vi "NATS SUB.vi"(6 "timeout ms (conn default)":i32=-2, 7 "queue group":string, 8 "error in":errorcluster caption="error in (no error)", 9 "subject":string, 10 "sub id":string, 11 "nats connection in":T1={"connection ID"=refnum, "server INFO"="", "timeout ms"=5000, "verbose?"=FALSE, "server headers?"=FALSE, "client headers?"=FALSE}) -> (0 "error out":errorcluster, 2 "dup sub id":string, 3 "dup nats connection":T1={"connection ID"=refnum, "server INFO"="", "timeout ms"=5000, "verbose?"=FALSE, "server headers?"=FALSE, "client headers?"=FALSE})   [LabVIEW 2013, in "NATS Core.lvlib"]
doc: "Subscribes to a NATS subject with the specified subscription ID."
uses:
  NATS Core.lvlib
  Controls/nats connection.ctl
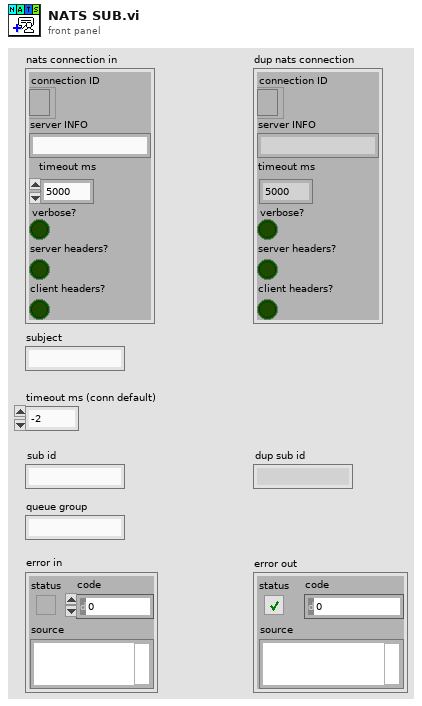
[diagram p1: front panel]
types:
  T1 = typedef "NATS Core.lvlib/nats connection.ctl" = cluster{"connection ID":refnum<k5>, "server INFO":string, "timeout ms":i32, "verbose?":bool, "server headers?":bool, "client headers?":bool}
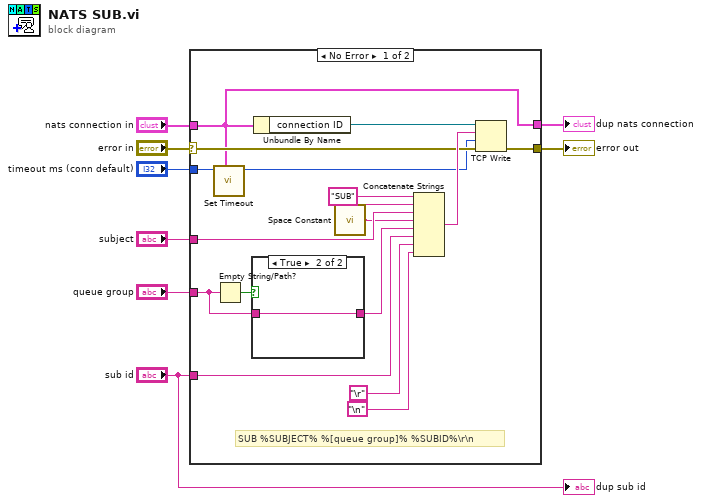
[diagram p0: block diagram]
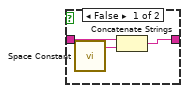
[diagram p2: hidden frame]
diagram:
  n1 = case shown="No Error" "error in" {
    selector: "error in" -> [w15 w30]
    tunnel: "nats connection in" -> [w14 w29]
    tunnel: [w23 w30] -> w7
    tunnel: "timeout ms (conn default)" -> [w13 _]
    tunnel: "subject" -> [w21 _]
    tunnel: "sub id" -> [w19 _]
    tunnel: [w14 w29] -> w2
    tunnel: "queue group" -> [w10 _]
    frame No Error {
      # "SUB %SUBJECT% %[queue group]% %SUBID%\\r\\n"
      n2 = call "Set Timeout.vi"("nats connection in"=w14, "timeout ms in"=w13) -> ("timeout ms out"=w12:i32)  [unwired: 9 in]
      n3 = Empty String/Path?(string/path=w10) -> (empty?=w11:bool)
      n4 = case shown="True" w11 {
        tunnel: w10 -> [w27 w28]
        tunnel: [w25 w28] -> w9
        frame False {
          n5 = call <vilib>:"Space Constant.vi"() -> ("String"=w26:string)
          n6 = Concatenate Strings(w27, w26) -> (w25:string)
        }
        frame True {
        }
      }
      n7 = Unbundle By Name(w14) -> ("connection ID"=w24:refnum<k5>)
      n8 = call <vilib>:"Space Constant.vi"() -> ("String"=w20:string)
      n9 = Concatenate Strings("SUB" ("string"), w20, w21, w20, w9, w19, "\r", "\n") -> (w16:string)
      n10 = TCP Write(connection ID=w24, data in=w16, error in (no error)=w15, 9:w12) -> (error out=w23:errorcluster)  [unwired: 2 out]
    }
    frame Error {
    }
  }
  "error out" <- w7
  "dup nats connection" <- w2
  "dup sub id" <- "sub id"
